vi "Save to File.vi"(7 "Replace if Exists? (F)":bool, 8 "error in (no error)":errorcluster, 10 "Maze File Path (*.maz)":path, 11 "Maze In":refnum<class "Maze.lvclass">) -> (0 "error out":errorcluster, 3 "Maze":refnum<class "Maze.lvclass">)   [LabVIEW 2020, in "App.lvlib" / "MazeFileIO.lvclass"]
uses:
  MazeFileIO.lvclass
  Maze/Maze/Maze.lvclass
  Maze/Maze/Get Goal.vi
  Maze/Maze/Get Start.vi
  Maze/Maze/Get Adjacency.vi
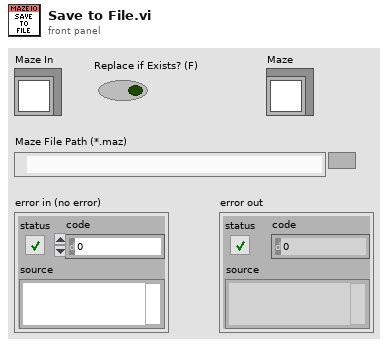
[diagram p1: front panel]
types:
  T1 = enum16{"open", "replace", "create", "open or create", "replace or create", "replace or create with confirmation"}
  T2 = typedef "Maze.lvlib/Position.ctl" = cluster{"S":i32, "E":i32}
  T3 = typedef "Maze.lvlib/Adjacency.ctl" = cluster{"E":bool, "N":bool, "W":bool, "S":bool, "Goal":bool, "Start":bool}
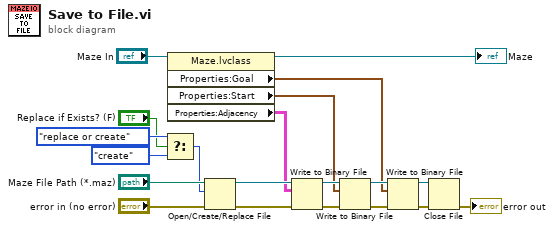
[diagram p0: block diagram]
diagram:
  n1 = Select(t=T1."replace or create" ("operation (0:open)"), s="Replace if Exists? (F)", f=T1."create") -> (s? t:f=w15:T1)
  n2 = property class="Maze.lvclass"(reference="Maze In") -> (reference out=→"Maze":refnum<class "Maze.lvclass">, "Properties:Goal"=w1:T2, "Properties:Start"=w2:T2, "Properties:Adjacency"=w10:T3[][])  [unwired: 1 in, 1 out]
  n3 = Open/Create/Replace File(file path (use dialog)="Maze File Path (*.maz)", error in="error in (no error)", operation (0:open)=w15) -> (refnum out=w12:refnum<file>, error out=w11:errorcluster)  [unwired: 3 in, 1 out]
  n4 = Write to Binary File(file (use dialog)=w12, data=w10, error in=w11) -> (refnum out=w9:refnum<file>, error out=w8:errorcluster)  [unwired: 3 in, 1 out]
  n5 = Write to Binary File(file (use dialog)=w9, data=w2, error in=w8) -> (refnum out=w6:refnum<file>, error out=w7:errorcluster)  [unwired: 3 in, 1 out]
  n6 = Write to Binary File(file (use dialog)=w6, data=w1, error in=w7) -> (refnum out=w4:refnum<file>, error out=w5:errorcluster)  [unwired: 3 in, 1 out]
  n7 = Close File(refnum=w4, error in=w5) -> (error out=→"error out":errorcluster)  [unwired: 1 out]
